vi "Scale X And A B Mode.vi"(0 "VISA resource name":refnum<visa-resource-name>, 1 "Maximum A (1.0E+6)":dbl=1000000.0 min=-9.999e+37 max=9.99e+37 format="%^.3e", 2 "Minimum A (0.0)":dbl min=-9.999e+37 max=1e+38 format="%^.3e", 3 "Scale A (0:Autoscale)":u32(ring) items=["Autoscale", "Min/Max", "Scale Division"], 5 "Scale Division A (5.0E-3)":dbl=0.005 min=5e-36 max=9.999e+36 format="%^.3e", 7 "Scale B (0:Autoscale)":u32(ring) items=["Autoscale", "Min/Max", "Scale Division"], 9 "Minimum B (0.0)":dbl min=-1e+38 max=9.99e+37 format="%^.3e", 11 "error in (no error)":errorcluster, 12 "Maximum B (1.0E+6)":dbl=1000000.0 min=-9.999e+37 max=9.99e+37 format="%^.3e", 13 "Scale Division B (5.0E-3)":dbl=0.005 min=5e-36 max=9.999e+36 format="%^.3e") -> (4 "VISA resource name out":refnum<visa-resource-name>, 15 "error out":errorcluster)   [LabVIEW 2011, in "Agilent 4194.lvlib"]
doc: "This function sets the display scale parameters effective for X - A&B.\n\nNotes:\n\n(1) This function is valid for X - A&B setting only."
uses:
  <instrlib>/Agilent 4194/Agilent 4194.lvlib
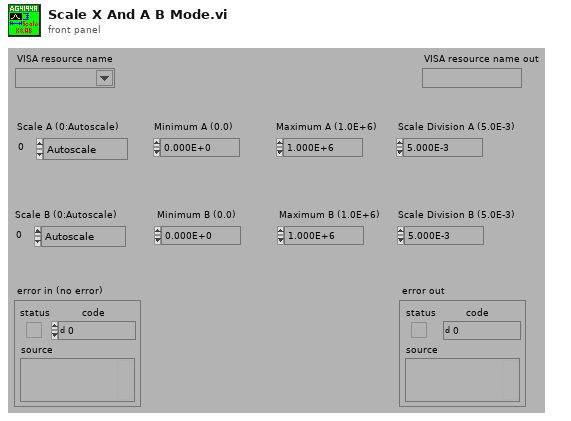
[diagram p1: front panel]
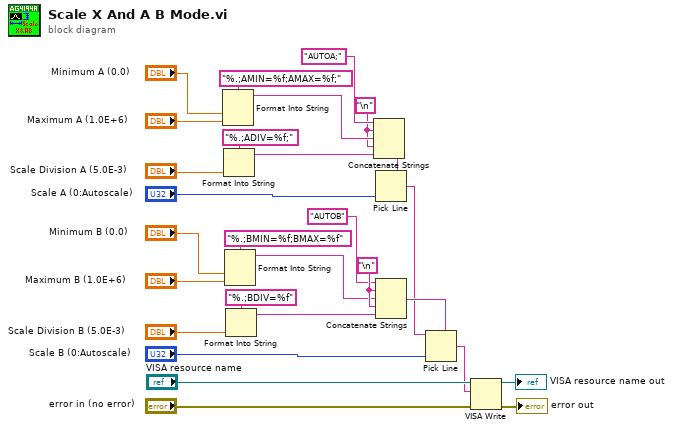
[diagram p0: block diagram]
diagram:
  w16 = "\n"
  w20 = "\n"
  n1 = Format Into String(format string="%.;AMIN=%f;AMAX=%f;", "Minimum A (0.0)", "Maximum A (1.0E+6)") -> (resulting string=w22:string)  [unwired: 2 in, 1 out]
  n2 = Format Into String(format string="%.;ADIV=%f;", "Scale Division A (5.0E-3)") -> (resulting string=w21:string)  [unwired: 2 in, 1 out]
  n3 = Format Into String(format string="%.;BMIN=%f;BMAX=%f", "Minimum B (0.0)", "Maximum B (1.0E+6)") -> (resulting string=w14:string)  [unwired: 2 in, 1 out]
  n4 = Format Into String(format string="%.;BDIV=%f", "Scale Division B (5.0E-3)") -> (resulting string=w15:string)  [unwired: 2 in, 1 out]
  n5 = Concatenate Strings("AUTOA;", w20, w22, w20, w21) -> (w19:string)
  n6 = Pick Line(multi-line string=w19, line index="Scale A (0:Autoscale)") -> (output string=w6:string)  [unwired: 1 in]
  n7 = Concatenate Strings("AUTOB", w16, w14, w16, w15) -> (w17:string)
  n8 = Pick Line(string ("")=w6, multi-line string=w17, line index="Scale B (0:Autoscale)") -> (output string=w1:string)
  n9 = VISA Write(VISA resource name="VISA resource name", write buffer=w1, error in (no error)="error in (no error)") -> (VISA resource name out=→"VISA resource name out":refnum<visa-resource-name>, error out=→"error out":errorcluster)  [unwired: 1 out]
